vi "artInitParm.vi"() -> (0 "待读取长度":dbl, 1 "量程选择":dbl, 2 "初始化参数":dbl[](array[numeric]))   [LabVIEW 2018]
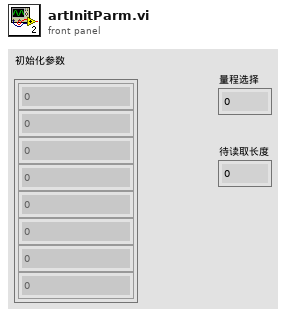
[diagram p1: front panel]
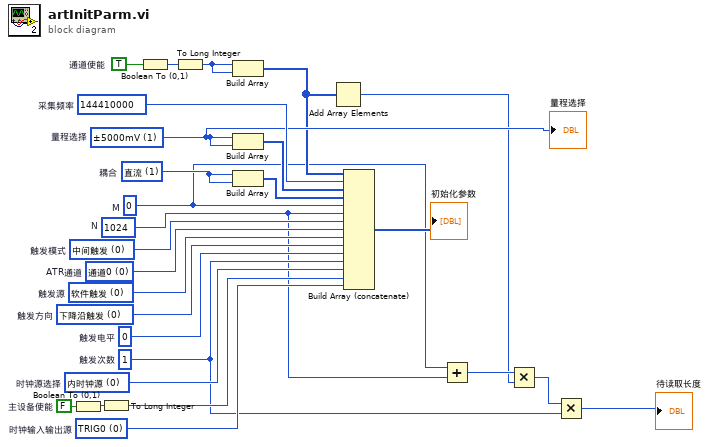
[diagram p0: block diagram]
diagram:
  w1 = 1024  # N
  w2 = 0  # M
  w12 = 1 items=["交流", "直流"]  # 耦合
  w9 = 1 items=["±1000mV", "±5000mV"]  # 量程选择
  w14 = TRUE  # 通道使能
  w11 = 144410000  # 采集频率
  w17 = 0 items=["中间触发", "后触发", "预触发", "硬件延时触发"]  # 触发模式
  w15 = 0 items=["通道0", "通道1"]  # ATR通道
  w25 = 0 items=["软件触发", "DTR作为触发源", "ATR作为触发源", "Trigger信号触发"]  # 触发源
  w24 = 0 items=["下降沿触发", "上升沿触发", "上下边沿均触发", ""]  # 触发方向
  w23 = 0  # 触发电平
  w5 = 1  # 触发次数
  w21 = 0 items=["TRIG0", "TRIG1", "TRIG2", "TRIG3"]  # 时钟输入输出源
  w27 = FALSE  # 主设备使能
  w22 = 0 items=["内时钟源", "主卡10M时钟源", "外部时钟"]  # 时钟源选择
  n1 = Boolean To (0,1) ("布尔值至(0,1)转换")(Boolean=w27) -> (0, 1=w19:i16)
  n2 = To Long Integer(number=w19) -> (32bit integer=w20:i32)
  n3 = Boolean To (0,1)(Boolean=w14) -> (0, 1=w18:i16)
  n4 = To Long Integer(number=w18) -> (32bit integer=w13:i32)
  n5 = Build Array(w13, w13) -> (w4:i32[])
  n6 = Build Array(w9, w9) -> (w16:i32[])
  n7 = Build Array(w12, w12) -> (w26:i32[])
  n8 = Add Array Elements(numeric array=w4) -> (sum=w3:i32)
  n9 = Build Array (concatenate) ("创建数组")(w4, w11, w16, w26, w2, w1, w17, w15, w25, w24, w23, w5, w22, w20, w21) -> (→"初始化参数":i32[])
  n10 = Add(x=w2, y=w1) -> (x+y=w8:i32)
  n11 = Multiply(x=w8, y=w3) -> (x*y=w7:i32)
  n12 = Multiply(x=w7, y=w5) -> (x*y=→"待读取长度":i32)
  "量程选择" <- w9
